vi "CameraGetValueAttr.vi"(8 "error in":errorcluster, 10 "Attr String":string, 11 "IMAQdx Session In":T1) -> (0 "error out":errorcluster, 1 "Auto?":bool, 2 "Value":string="Manual", 3 "IMAQdx Session out":T1)   [LabVIEW 2025]
doc: "Set the Mode of the attribute to Manual or Auto.\n\nThis software is licensed. Open the labview\\readme\\WPI Robotics Library Open Source License.txt file for more information."
uses:
  <vilib>/userDefined/High Color/IMAQdx.ctl
  <resource>/objmgr/imaqdx.rc
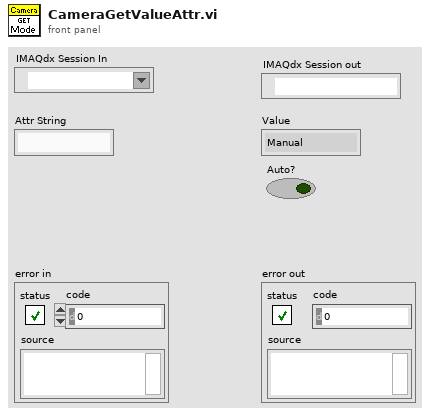
[diagram p1: front panel]
types:
  T1 = typedef "IMAQdx.ctl" = refnum<k21>
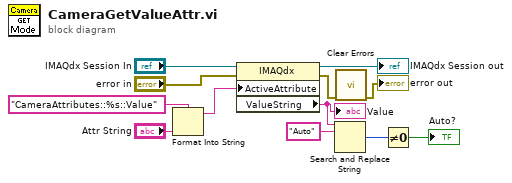
[diagram p0: block diagram]
diagram:
  n1 = Format Into String(format string="CameraAttributes::%s::Value" ("Attr Format"), "Attr String") -> (resulting string=w11:string)  [unwired: 2 in, 1 out]
  n2 = property class="IMAQdx"(reference="IMAQdx Session In", error in="error in", "ActiveAttribute"=w11) -> (reference out=→"IMAQdx Session out":T1, error out=w9:errorcluster, "ValueString"=w1:string)
  "Value" <- w1
  n3 = Search and Replace String(input string=w1, search string="Auto") -> (number of replacements=w3:i32)  [unwired: 6 in, 3 out]
  n4 = call <vilib>:"Clear Errors.vi"("error in (no error)"=w9) -> ("error out"=→"error out":errorcluster)  [unwired: 5 in, 1 out]
  n5 = Not Equal To 0?(x=w3) -> (x != 0?=→"Auto?":bool)
